vi "Measurement UI.vi"() -> ()   [LabVIEW 2025, in "Workflow DO UI.lvlib"]
uses:
  Workflow DO UI.lvlib
panel:
  out "CAN Error":bool
  out "Message Buffer":string[][](table)
  in  "TYPE":u32(ring) items=["CAN Data"=0, "CAN Remote"=1, "CAN Bus Error"=2, "CAN 2.0 Data"=8, "CAN FD Data"=16, "CAN FD+BRS Data"=24, "J1939 Data"=192, "Delay"=224, "Log Trigger"=225, "Start Trigger"=226]
  in  "CAN Interface Name":string
  in  "Termination CAN":bool
  out "Timeout":bool
  out "Count":u32
  out "Trace":string[][](table)
  out "Digital Input":u32[](graph)
  in  "IO Mode":enum32{"CAN", "CAN FD", "CAN FD + BRS"}(ring)
  in  "FD ISO Mode":enum32{"ISO", "Legacy ISO", "Non-ISO"}(ring)=enum."Non-ISO"
  in  "Baudrate":u32=125000 format="%x"
  in  "FD Baudrate":u32 format="%x"
  in  "INTERFACE NAME CAN":refnum<k21>="CAN1"
  in  "PAYLOAD":u32[](array[numeric])=[0, 1, 2, 3, 4, 5, 6, 7] format="%x"
  in  "IDENTIFIER":u32=1034 format="%x"
  in  "Timeout (s)":u32=30
  in  "Pulses":u32=20
  in  "Counter Interface":string
  in  "Input Terminal Name":string
  in  "Active Edge":i32(ring)=10171 items=["Rising"=10280, "Falling"=10171]
  in  "Input Terminal":tag="/PXI1Slot6/PFI0"
  in  "Counter":tag="PXI1Slot6/ctr0"
  # "Digital Channel Settings"
  # "CAN Settings"
  # "Number of Expected Pulses"
  # "CAN Trace"
  # "Results"
  # "Counter"
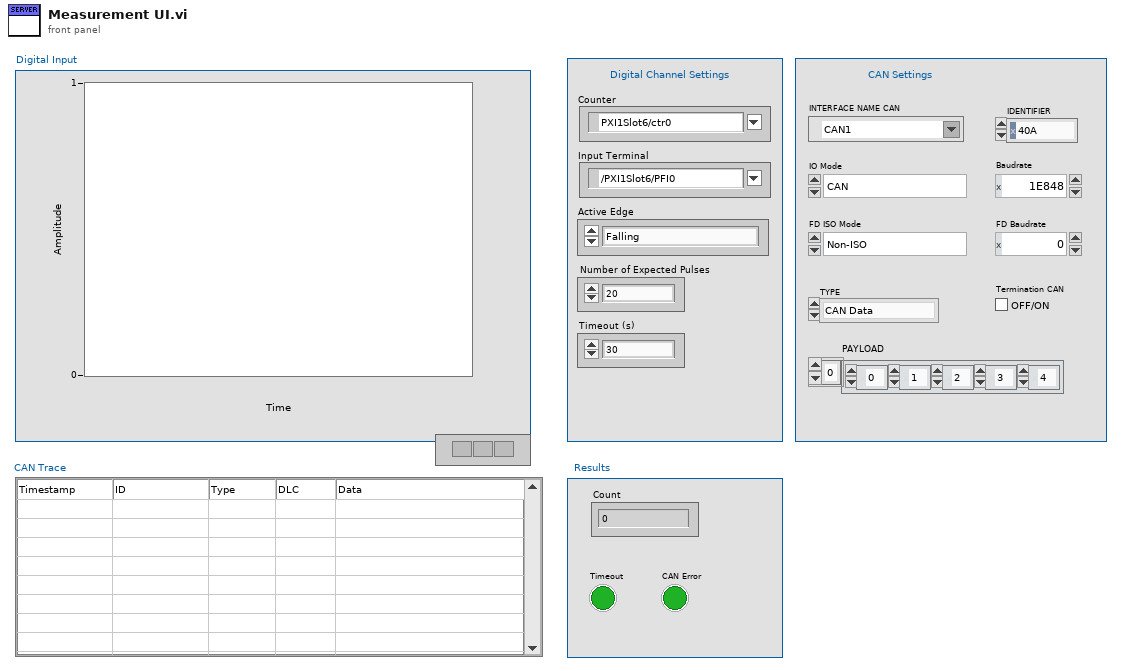
[diagram p1: front panel]
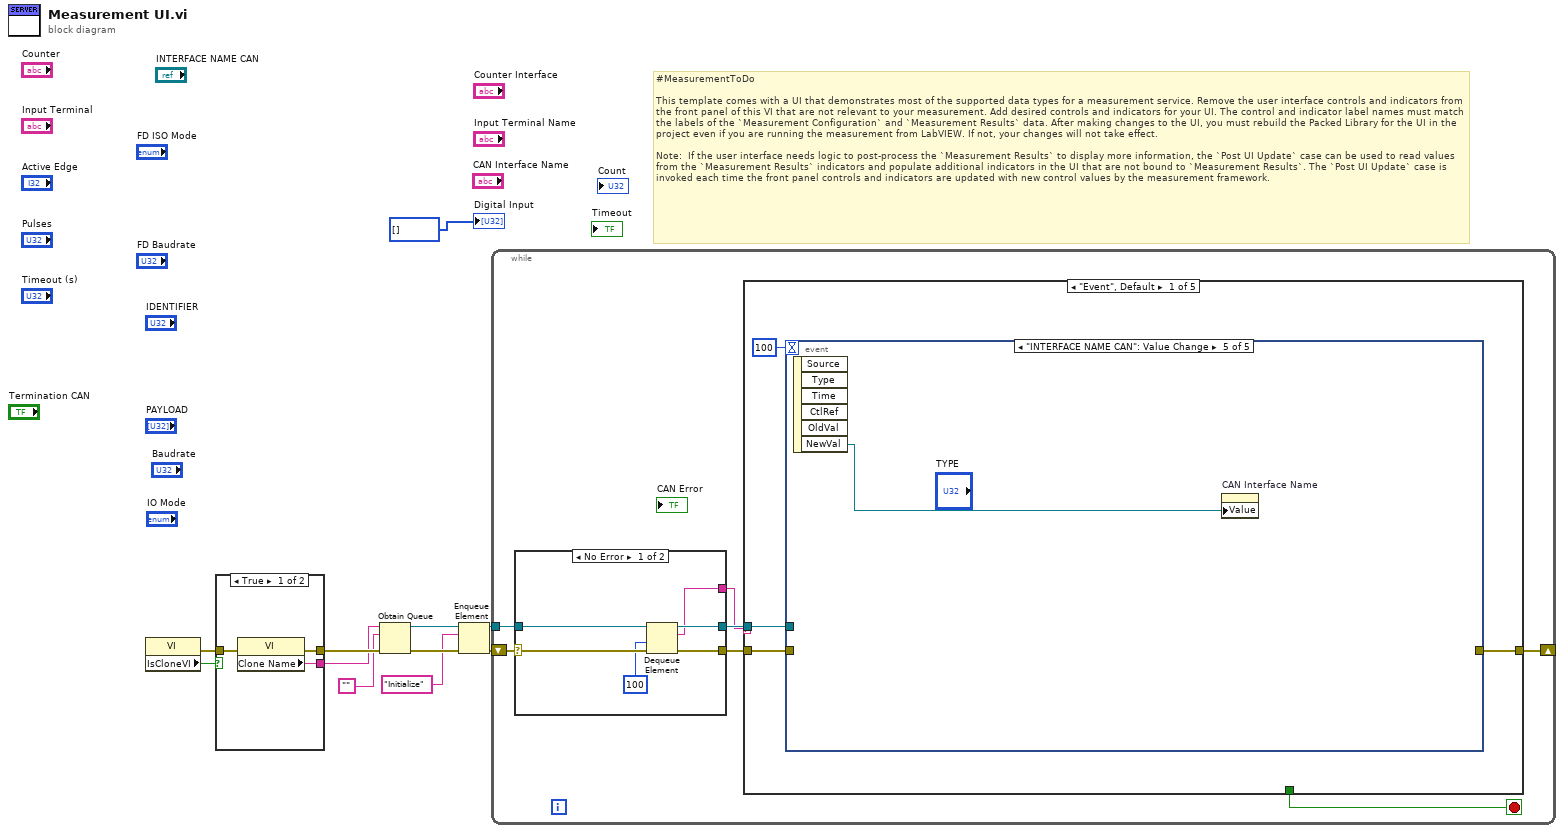
[diagram p0: block diagram]
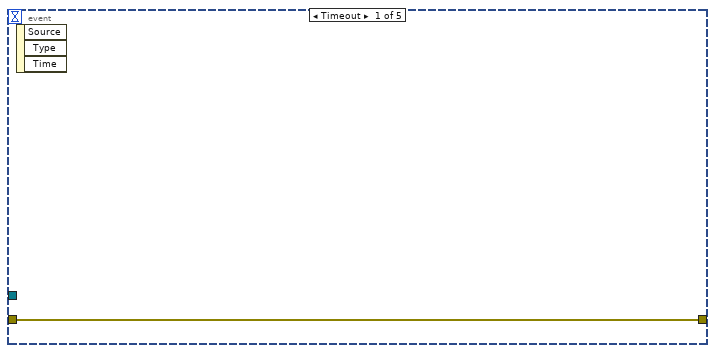
[diagram p2: hidden frame]
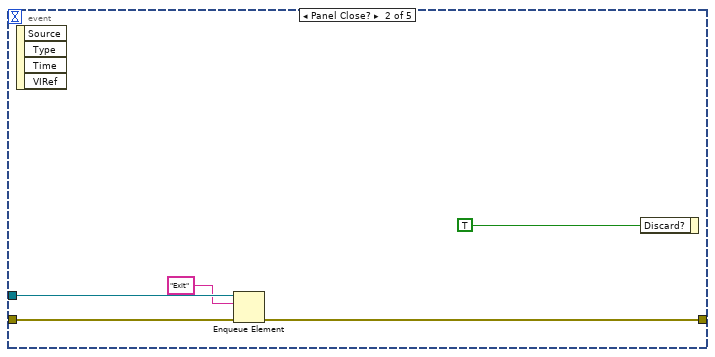
[diagram p3: hidden frame]
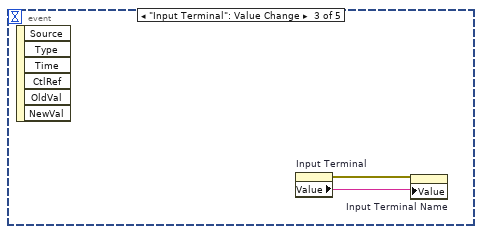
[diagram p4: hidden frame]
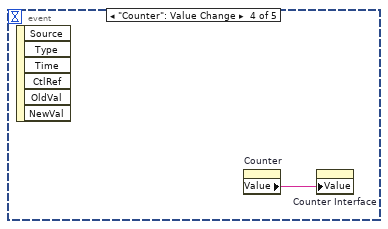
[diagram p5: hidden frame]
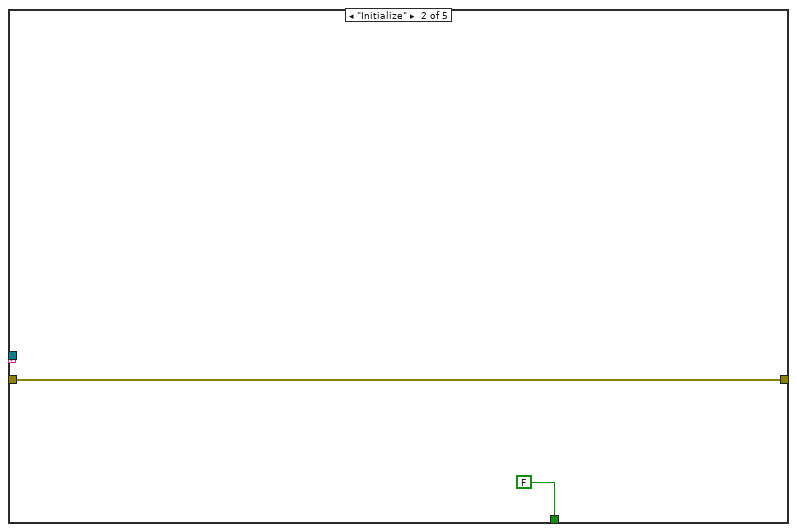
[diagram p6: hidden frame]
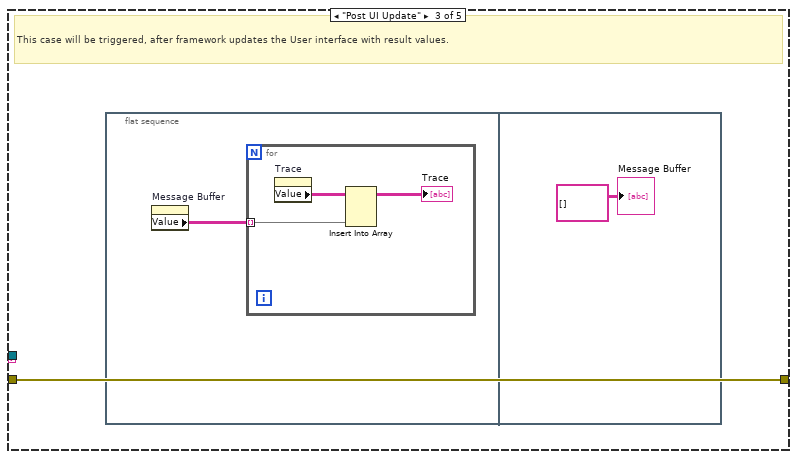
[diagram p7: hidden frame]
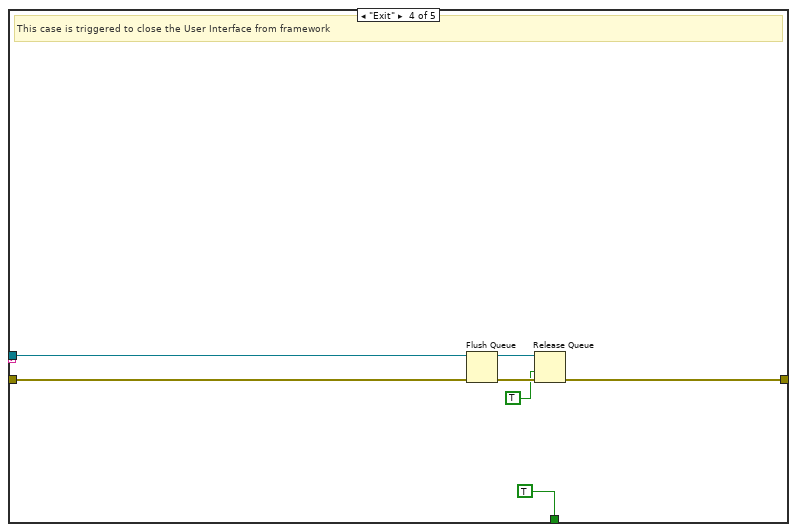
[diagram p8: hidden frame]
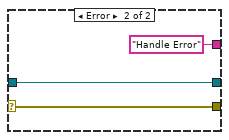
[diagram p10: hidden frame]
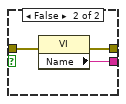
[diagram p11: hidden frame]
diagram:
  # "#MeasurementToDo  \n\nThis template comes with a UI that demonstrates most of the supported data types for a measurement service. Remove the user interface controls and indicators from the front panel of this VI that are not relevant to your measurement. Add desired controls and indicators for your UI. The control and indicator label names must match the labels of the `Measurement Configuration` and `Measurement Results` data. After making changes to the UI, you must rebuild the Packed Library for the UI in the project even if you are running the measurement from LabVIEW. If not, your changes will not take effect.\n\nNote:  If the user interface needs logic to post-process the `Measurement Results` to display more information, the `Post UI Update` case can be used to read values from the `Measurement Results` indicators and populate additional indicators in the UI that are not bound to `Measurement Results`. The `Post UI Update` case is invoked each time the front panel controls and indicators are updated with new control values by the measurement framework."
  n1 = property class="VI"() -> (error out=w2:errorcluster, "IsCloneVI"=w3:bool)  [unwired: 2 in, 1 out]
  n2 = case shown="True" w3 {
    tunnel: [w14 w17] -> w11
    tunnel: [w13 w16] -> w10
    tunnel: w2 -> [w12 w15]
    frame True {
      n3 = property class="VI"(error in=w12) -> (error out=w14:errorcluster, "Clone Name"=w13:string)  [unwired: 1 in, 1 out]
    }
    frame False {
      n4 = property class="VI"(error in=w15) -> (error out=w17:errorcluster, "Name"=w16:string)  [unwired: 1 in, 1 out]
    }
  }
  n5 = Obtain Queue(name (unnamed)=w10, element data type="", error in (no error)=w11) -> (queue out=w7:refnum<queue>, error out=w9:errorcluster)  [unwired: 2 in, 1 out]
  n6 = Enqueue Element(queue=w7, element="Initialize", error in (no error)=w9) -> (queue out=w6:refnum<queue>, error out=w8:errorcluster)  [unwired: 1 in, 1 out]
  n7 = while {
    shift-right: [w19] -> _
    shift-left: w8 -> [w24]
    tunnel: w6 -> [w22]
    stop <- w18 stop-if-true
    n8 = case shown="No Error" w24 {
      selector: w24 -> [w60 w63]
      tunnel: [w59 w63] -> w23
      tunnel: w22 -> [w58 w62]
      tunnel: [w57 w62] -> w21
      tunnel: [w56 "Handle Error"] -> w20
      frame No Error {
        n9 = Dequeue Element(queue=w58, timeout in ms (-1)=100, error in (no error)=w60) -> (queue out=w57:refnum<queue>, element=w56:string, error out=w59:errorcluster)  [unwired: 1 out]
      }
      frame Error {
      }
    }
    n10 = case shown="\"Event\", Default" w20 {
      tunnel: w23 -> [w27 w40 w41 w53 w54]
      tunnel: w21 -> [w25 _ _ w51 _]
      tunnel: [w28 w40 w41 w48 w54] -> w19
      tunnel: [_ FALSE _ TRUE _] -> w18
      frame "Event", Default {
        n11 = event shown="[4] \"INTERFACE NAME CAN\": Value Change" {
          selector: _ -> [_ _ _ _ _]
          dyn-events: _ -> [_ _ _ _ _]
          timeout: 100 -> [_ _ _ _ _]
          tunnel: [w29 w32 _ _ _] -> w28
          tunnel: w27 -> [w29 w33 _ _ _]
          tunnel: w25 -> [_ w31 _ _ _]
          event Timeout {
            n12 = event-data() -> ()  [unwired: 1 in, 3 out]
          }
          event Panel Close? {
            n13 = event-data() -> ()  [unwired: 1 in, 4 out]
            n14 = Enqueue Element(queue=w31, element="Exit", error in (no error)=w33) -> (error out=w32:errorcluster)  [unwired: 1 in, 2 out]
            n15 = event-data("Discard?"=TRUE) -> ()  [unwired: 1 in, 1 out]
          }
          event "Input Terminal": Value Change {
            n16 = event-data() -> ()  [unwired: 1 in, 6 out]
            n17 = property on="Input Terminal" class="DAQmxName"() -> (error out=w35:errorcluster, "Value"=w36:string)  [unwired: 2 in, 1 out]
            n18 = property on="Input Terminal Name" class="Str"(error in=w35, "Value"=w36) -> ()  [unwired: 1 in, 2 out]
          }
          event "Counter": Value Change {
            n19 = event-data() -> ()  [unwired: 1 in, 6 out]
            n20 = property on="Counter" class="DAQmxName"() -> ("Value"=w37:string)  [unwired: 2 in, 2 out]
            n21 = property on="Counter Interface" class="Str"("Value"=w37) -> ()  [unwired: 2 in, 2 out]
          }
          event "INTERFACE NAME CAN": Value Change {
            n22 = event-data() -> ("NewVal"=w38:refnum<k21>)  [unwired: 1 in, 5 out]
            n23 = property on="CAN Interface Name" class="Str"("Value"=w38) -> ()  [unwired: 2 in, 2 out]
          }
        }
      }
      frame "Initialize" {
      }
      frame "Post UI Update" {
        # "This case will be triggered, after framework updates the User interface with result values."
        n24 = flat-sequence {
          frame #0 {
            n25 = property on="Message Buffer" class="Tbl (strict)"() -> ("Value"=w42:string[][])  [unwired: 2 in, 2 out]
            n26 = for {
              tunnel: w42 -> [w44] mode=indexing
              n27 = property on="Trace" class="Tbl (strict)"() -> ("Value"=w45:string[][])  [unwired: 2 in, 2 out]
              n28 = Insert Into Array(array=w45, new element=w44) -> (→"Trace":string[][])  [unwired: 2 in]
            }
          }
          frame #1 {
            "Message Buffer" <- string[][] [] ("Message Buffer")
          }
        }
      }
      frame "Exit" {
        # "This case is triggered to close the User Interface from framework"
        n29 = Flush Queue(queue=w51, error in (no error)=w53) -> (queue out=w50:refnum<queue>, error out=w49:errorcluster)  [unwired: 1 out]
        n30 = Release Queue(queue=w50, force destroy? (F)=TRUE, error in (no error)=w49) -> (error out=w48:errorcluster)  [unwired: 2 out]
      }
      frame "Handle Error" {
      }
    }
  }
  "Digital Input" <- u32[] []
